vi "Write 02-06-9265 Vals.vi"(8 "error in (no error)":errorcluster, 11 "Data (4Channs AO) (Empty: Default)":dbl[](array[numeric])) -> (0 "error out":errorcluster)   [LabVIEW 2018, in "Outputs.lvlib"]
doc: "This subVI enqueues the named action in to the communications queue along with the input data."
uses:
  Outputs.lvlib
  Private Controls/Module Data.ctl
  Private Controls/Module Action.ctl
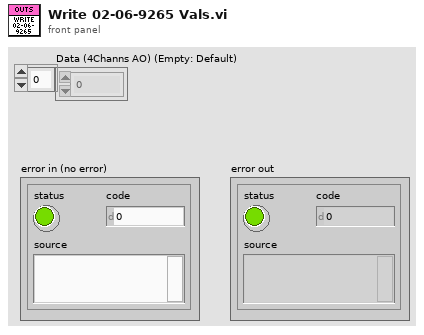
[diagram p1: front panel]
types:
  T1 = typedef "Outputs.lvlib/Module Data.ctl" = cluster{"Data":variant, "Action":T2}
  T2 = typedef "Outputs.lvlib/Module Action.ctl" = enum16{"Init", "Error", "StartStop Acquisition", "Write 02-06-9265 Vals (AO)", "Write 00-04-9265 Vals (AO)", "Write 02-00-9485 Vals (DO)", "Write 02-01-9485 Vals (DO)", "Set APU&ECU Cntrls", "Set Bleed-Fuel-ECS Cntrls", "Set ECS Demnd Cluster", "Set Fuel Pres Regltr", "Write Single 02-00-9485 Chann", "Write Single 02-01-9485 Chann", "Write Single 00-04-9265 Chann", "Set Sample Rate", "ESTOP"}
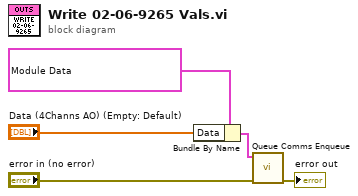
[diagram p0: block diagram]
diagram:
  n1 = Bundle By Name(cluster=T1 {"Data"=variant, "Action"=enum."Write 02-06-9265 Vals (AO)"} ("element"), "Data"="Data (4Channs AO) (Empty: Default)") -> (w4:T1)
  n2 = call "Queue Comms Enqueue.vi"("error in (no error)"="error in (no error)", "element"=w4) -> ("error out"=→"error out":errorcluster)  [unwired: 9 in]
